vi "Untitled 6 (SubVI).vi"(11 "celsius":dbl) -> (3 "Numeric":dbl)   [LabVIEW 2020]
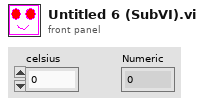
[diagram p1: front panel]
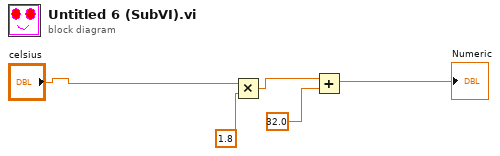
[diagram p0: block diagram]
diagram:
  n1 = Multiply(x="celsius", y=1.8) -> (x*y=w2:dbl)
  n2 = Add(x=w2, y=32.0) -> (x+y=→"Numeric":dbl)
